vi "makeDefaultFile.vi"(7 "utf-8":bool, 8 "에러 입력":errorcluster, 10 "생성 파일":cluster{"subject":string, "content":string}[](array[cluster]), 11 "디렉토리":path) -> (0 "에러 출력":errorcluster, 3 "파일 경로":path[](array[path]))   [LabVIEW 2018]
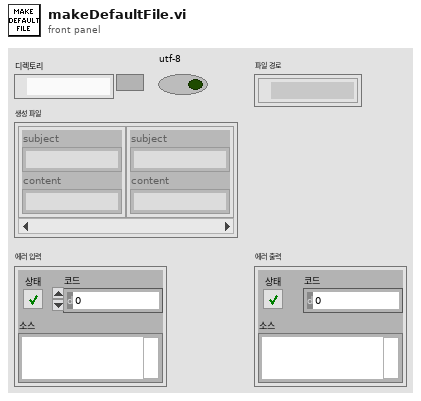
[diagram p1: front panel]
types:
  T1 = enum16{"open", "replace", "create", "open or create", "replace or create", "replace or create with confirmation"}
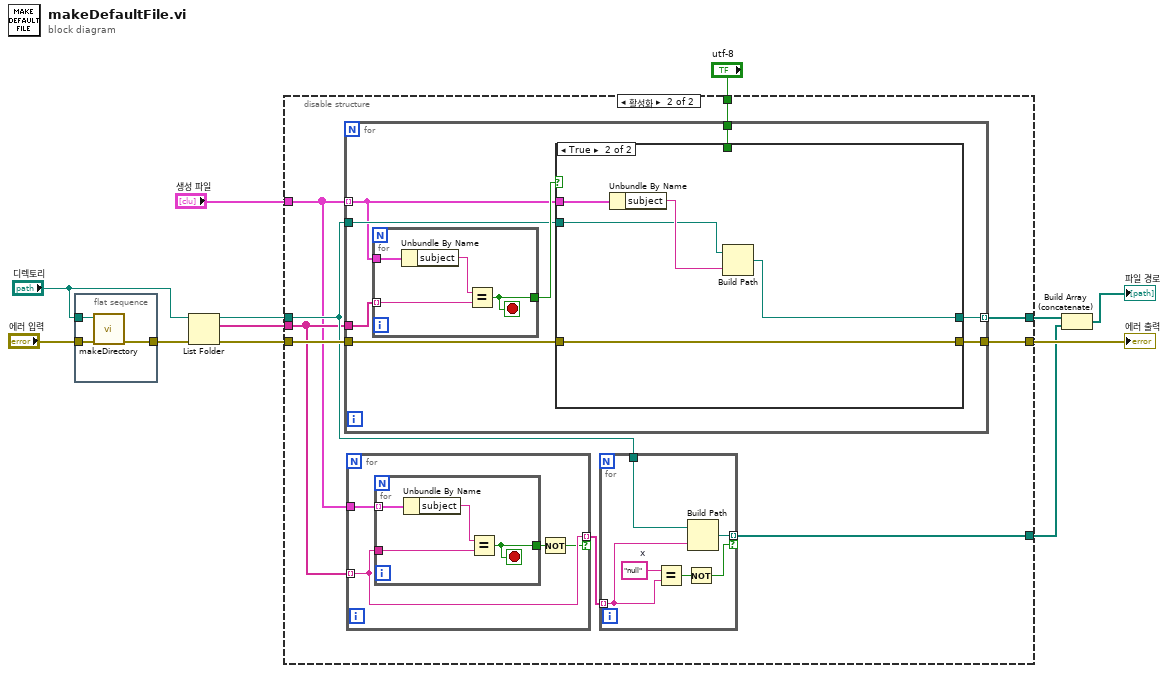
[diagram p0: block diagram]
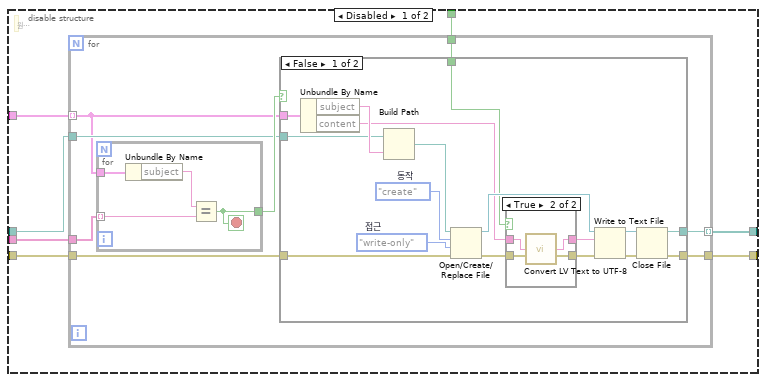
[diagram p2: hidden frame]
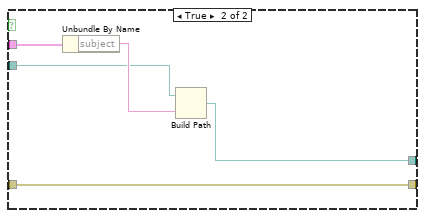
[diagram p4: hidden frame]
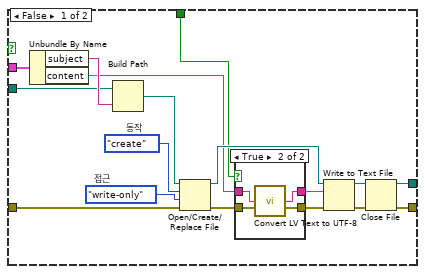
[diagram p5: hidden frame]
diagram:
  n1 = flat-sequence {
    tunnel: "디렉토리" -> [w15]
    tunnel: "에러 입력" -> [w14]
    tunnel: [w13] -> w12
    frame #0 {
      n2 = call "makeDirectory.vi"("error in"=w14, "파일저장경로"=w15) -> ("error out"=w13:errorcluster)  [unwired: 9 in]
    }
  }
  n3 = List Folder(path="디렉토리", error in=w12) -> (path out=w4:path, filenames=w6:string[], error out=w5:errorcluster)  [unwired: 2 in, 1 out]
  n4 = disable-structure shown="활성화" {
    disable-tunnel: "생성 파일" -> [w22 w64]
    disable-tunnel: [w21 w71] -> w3
    disable-tunnel: w4 -> [w20 w66]
    disable-tunnel: [w19 w70] -> w9
    disable-tunnel: w5 -> [w18 w69]
    disable-tunnel: w6 -> [w17 w65]
    disable-tunnel: "utf-8" -> [w16 w68]
    disable-tunnel: [_ w63] -> w1
    frame Disabled {
      # "원래 코드"
      n5 = for {
        tunnel: w17 -> [w30]
        tunnel: w22 -> [w24] mode=indexing
        tunnel: w18 -> [w28]
        tunnel: [w27] -> w19
        tunnel: w20 -> [w26]
        tunnel: [w25] -> w21 mode=indexing
        tunnel: w16 -> [w23]
        n6 = for {
          tunnel: w24 -> [w61]
          tunnel: w30 -> [w59] mode=indexing
          tunnel: [w62] -> w29
          stop <- w62 stop-if-true
          n7 = Unbundle By Name(w61) -> ("subject"=w60:string)
          n8 = Equal?(x=w60, y=w59) -> (x = y?=w62:bool)
        }
        n9 = case shown="False" w29 {
          tunnel: w24 -> [w42 w57]
          tunnel: [w44 w58] -> w27
          tunnel: w28 -> [w35 w58]
          tunnel: w26 -> [w37 w54]
          tunnel: [w39 w55] -> w25
          tunnel: w23 -> [w31 _]
          frame False {
            w40 = enum16{"read/write", "read-only", "write-only"}."write-only"  # 접근
            w41 = T1."create"  # 동작
            n10 = Unbundle By Name(w42) -> ("subject"=w38:string, "content"=w33:string)
            n11 = Build Path(base path=w37, name or relative path=w38) -> (appended path=w47:path)
            n12 = Open/Create/Replace File(file path (use dialog)=w47, error in=w35, operation (0:open)=w41, access (0:read/write)=w40) -> (refnum out=w46:refnum<file>, error out=w36:errorcluster)  [unwired: 2 in, 1 out]
            n13 = case shown="True" w31 {
              tunnel: w36 -> [w49 w50]
              tunnel: [w49 w51] -> w34
              tunnel: w33 -> [w48 w53]
              tunnel: [w48 w52] -> w32
              frame False {
              }
              frame True {
                n14 = call <vilib>:"Convert LV Text to UTF-8.vi"("LV Text"=w53, "error in"=w50) -> ("UTF-8 Text"=w52:string, "error out"=w51:errorcluster)  [unwired: 12 in]
              }
            }
            n15 = Write to Text File(file (use dialog)=w46, text=w32, error in=w34) -> (refnum out=w45:refnum<file>, error out=w43:errorcluster)  [unwired: 1 in, 1 out]
            n16 = Close File(refnum=w45, error in=w43) -> (path=w39:path, error out=w44:errorcluster)
          }
          frame True {
            n17 = Unbundle By Name(w57) -> ("subject"=w56:string)
            n18 = Build Path(base path=w54, name or relative path=w56) -> (appended path=w55:path)
          }
        }
      }
    }
    frame Enabled {
      n19 = for {
        tunnel: w65 -> [w93]
        tunnel: w64 -> [w87] mode=indexing
        tunnel: w69 -> [w91]
        tunnel: [w90] -> w70
        tunnel: w66 -> [w89]
        tunnel: [w88] -> w71 mode=indexing
        tunnel: w68 -> [w86]
        n20 = for {
          tunnel: w87 -> [w124]
          tunnel: w93 -> [w122] mode=indexing
          tunnel: [w125] -> w92
          stop <- w125 stop-if-true
          n21 = Unbundle By Name(w124) -> ("subject"=w123:string)
          n22 = Equal?(x=w123, y=w122) -> (x = y?=w125:bool)
        }
        n23 = case shown="True" w92 {
          tunnel: w87 -> [w105 w120]
          tunnel: [w107 w121] -> w90
          tunnel: w91 -> [w98 w121]
          tunnel: w89 -> [w100 w117]
          tunnel: [w102 w118] -> w88
          tunnel: w86 -> [w94 _]
          frame False {
            w103 = enum16{"read/write", "read-only", "write-only"}."write-only"  # 접근
            w104 = T1."create"  # 동작
            n24 = Unbundle By Name(w105) -> ("subject"=w101:string, "content"=w96:string)
            n25 = Build Path(base path=w100, name or relative path=w101) -> (appended path=w110:path)
            n26 = Open/Create/Replace File(file path (use dialog)=w110, error in=w98, operation (0:open)=w104, access (0:read/write)=w103) -> (refnum out=w109:refnum<file>, error out=w99:errorcluster)  [unwired: 2 in, 1 out]
            n27 = case shown="True" w94 {
              tunnel: w99 -> [w112 w113]
              tunnel: [w112 w114] -> w97
              tunnel: w96 -> [w111 w116]
              tunnel: [w111 w115] -> w95
              frame False {
              }
              frame True {
                n28 = call <vilib>:"Convert LV Text to UTF-8.vi"("LV Text"=w116, "error in"=w113) -> ("UTF-8 Text"=w115:string, "error out"=w114:errorcluster)  [unwired: 12 in]
              }
            }
            n29 = Write to Text File(file (use dialog)=w109, text=w95, error in=w97) -> (refnum out=w108:refnum<file>, error out=w106:errorcluster)  [unwired: 1 in, 1 out]
            n30 = Close File(refnum=w108, error in=w106) -> (path=w102:path, error out=w107:errorcluster)
          }
          frame True {
            n31 = Unbundle By Name(w120) -> ("subject"=w119:string)
            n32 = Build Path(base path=w117, name or relative path=w119) -> (appended path=w118:path)
          }
        }
      }
      n33 = for {
        tunnel: w65 -> [w79] mode=indexing
        tunnel: w64 -> [w81]
        tunnel: [w79] -> w67 mode=indexing if=w78
        n34 = for {
          tunnel: w81 -> [w84] mode=indexing
          tunnel: w79 -> [w82]
          tunnel: [w85] -> w80
          stop <- w85 stop-if-true
          n35 = Unbundle By Name(w84) -> ("subject"=w83:string)
          n36 = Equal?(x=w83, y=w82) -> (x = y?=w85:bool)
        }
        n37 = Not(x=w80) -> (.not. x?=w78:bool)
      }
      n38 = for {
        tunnel: w67 -> [w74] mode=indexing
        tunnel: w66 -> [w75]
        tunnel: [w73] -> w63 mode=indexing if=w72
        w76 = "null"  # x
        n39 = Equal?(x=w76, y=w74) -> (x = y?=w77:bool)
        n40 = Not(x=w77) -> (.not. x?=w72:bool)
        n41 = Build Path(base path=w75, name or relative path=w74) -> (appended path=w73:path)
      }
    }
  }
  "에러 출력" <- w9
  n42 = Build Array (concatenate)(w3, w1) -> (→"파일 경로":path[])
